vi "Process Mouse Move.vi"(0 "FSM.Graph in":T1, 5 "Display State In":T2, 7 "Coords":T3) -> (4 "FSM.Graph out":T1, 6 "Display State Out":T2, 10 "Refresh":bool)   [LabVIEW 2020, in "FSM Editor.xctl"]
uses:
  FSM Editor.xctl
  Classes/FSM.Graph/FSM.Graph.lvclass
  Classes/FSM.Port/FSM.Port.lvclass
  Drag Mode.ctl
  D:/Development/epl-vi-lib/Koop/KObject Class/KObject.lvclass
  D:/Development/epl-tosca/LV Source/FSM Graph VIs/LV Source/Classes/FSM.Graph/FSM.Graph.lvclass
  <vilib>/Utility/miscctls.llb/LVPoint32TypeDef.ctl
  State.vi
  Data.vi
  Events.ctl
  NodeAdded.ctl
  NodeSelected.ctl
  EdgeEventData.ctl
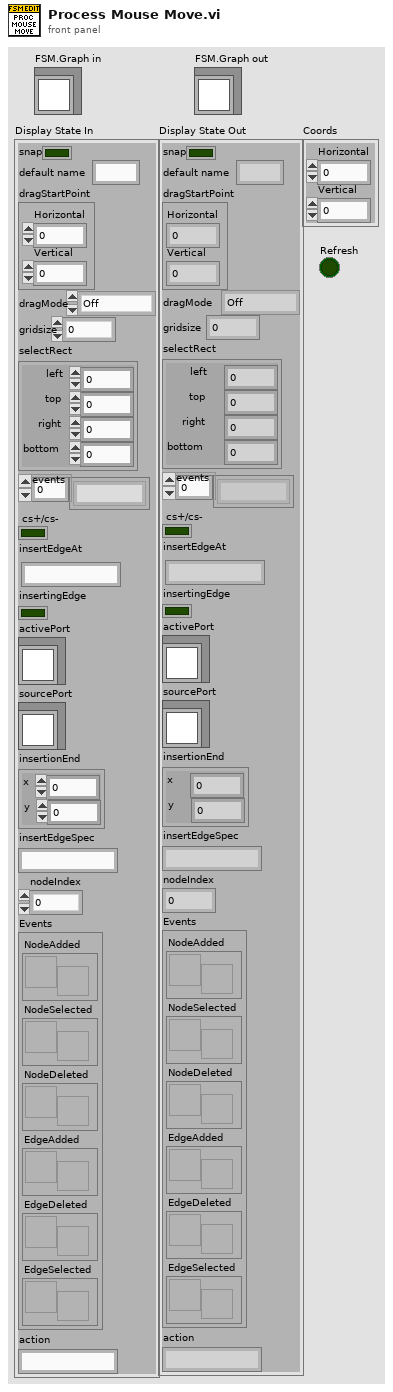
[diagram p1: front panel]
types:
  T1 = typedef "FSM Editor.xctl/Data.vi" = refnum<class "FSM.Graph.lvclass">
  T2 = typedef "FSM Editor.xctl/State.vi" = cluster{"snap":bool, "default name":string, "dragStartPoint":T3, "dragMode":T4, "gridsize":dbl, "selectRect":cluster{"left":i16, "top":i16, "right":i16, "bottom":i16}, "events":string[], "cs+/cs-":bool, "insertEdgeAt":string, "insertingEdge":bool, "activePort":refnum<class "FSM.Port.lvclass">, "sourcePort":refnum<class "FSM.Port.lvclass">, "insertionEnd":cluster{"x":i16, "y":i16}, "insertEdgeSpec":string, "nodeIndex":i32, "Events":T5, "action":string}
  T3 = typedef "LVPoint32TypeDef.ctl" = cluster{"Horizontal":i32, "Vertical":i32}
  T4 = typedef "Drag Mode.ctl" = enum16{"Off", "NodePending", "Nodes", "Pan", "Select", "EdgeInsertion", "EdgePoint", "EdgeLabel"}
  T5 = typedef "FSM Editor.xctl/Events.ctl" = cluster{"NodeAdded":refnum<user-event>, "NodeSelected":refnum<user-event>, "NodeDeleted":refnum<user-event>, "EdgeAdded":refnum<user-event>, "EdgeDeleted":refnum<user-event>, "EdgeSelected":refnum<user-event>}
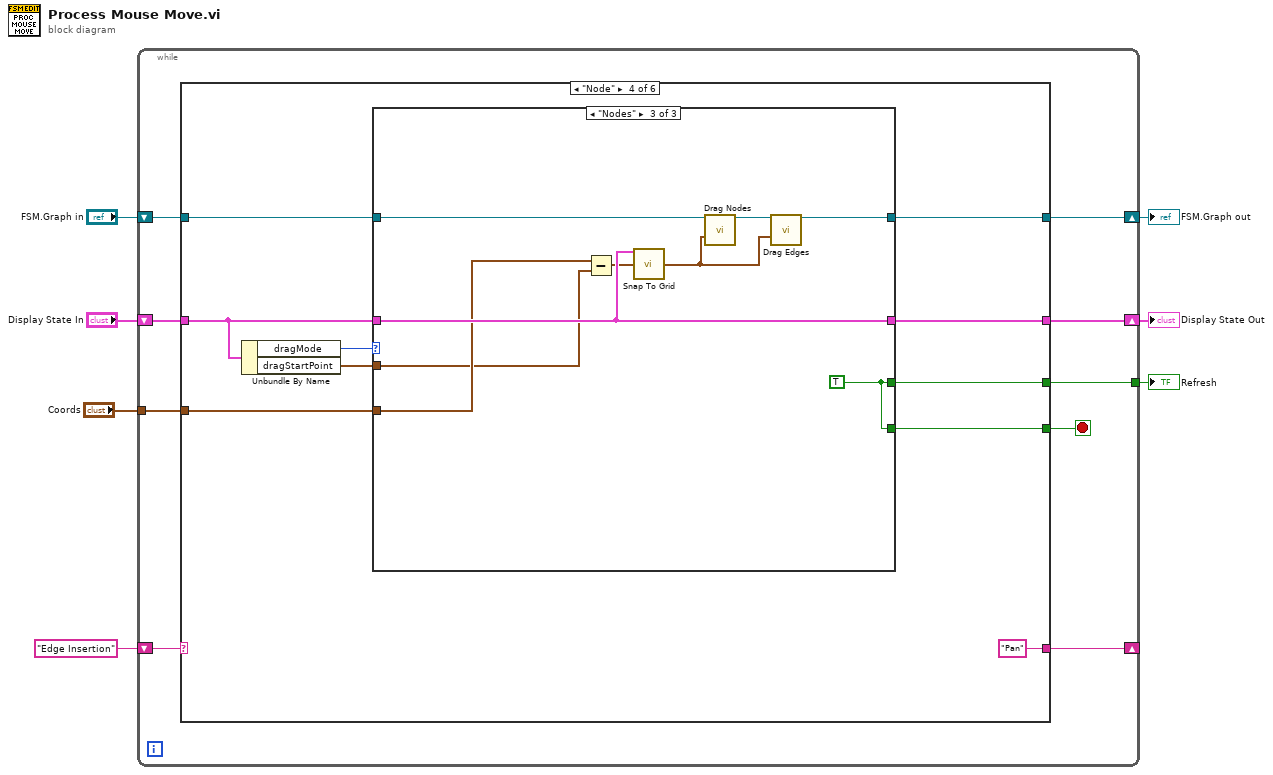
[diagram p0: block diagram]
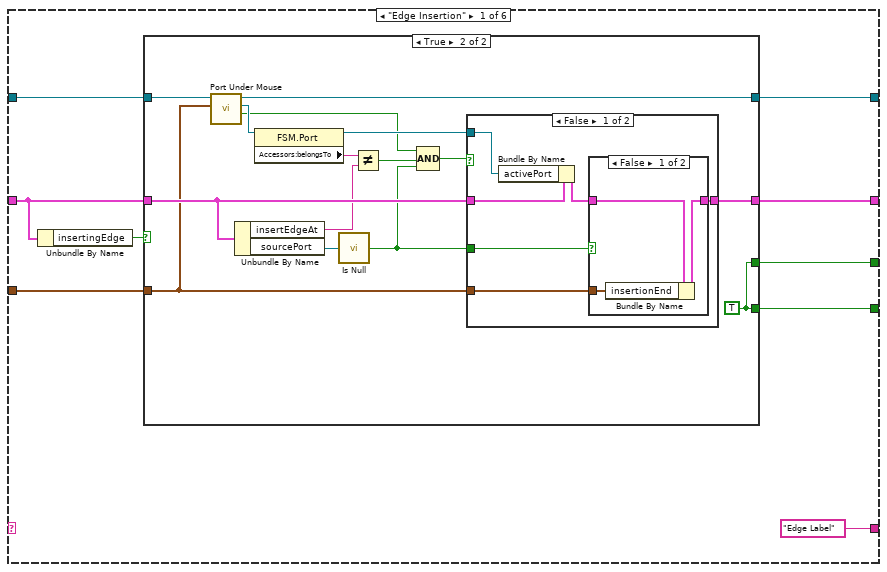
[diagram p2: hidden frame]
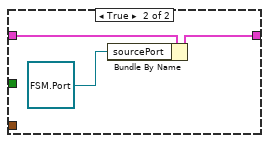
[diagram p5: hidden frame]
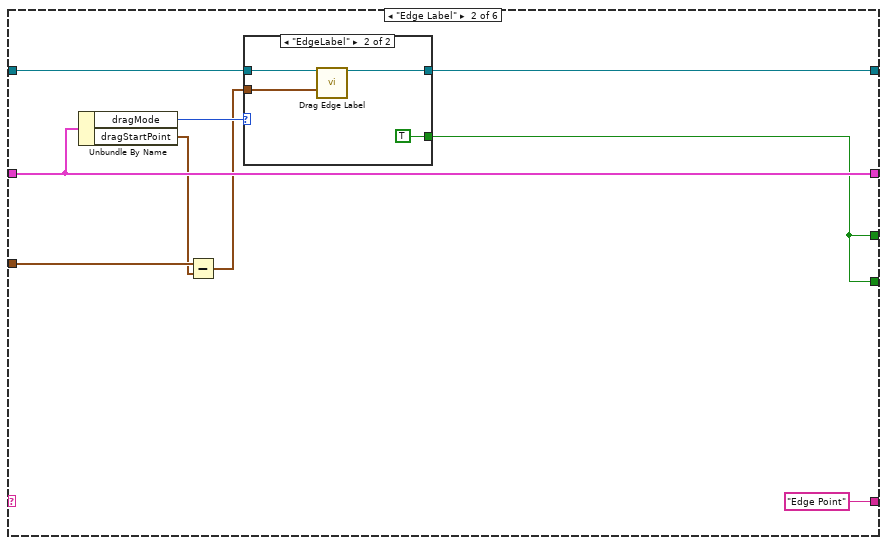
[diagram p6: hidden frame]
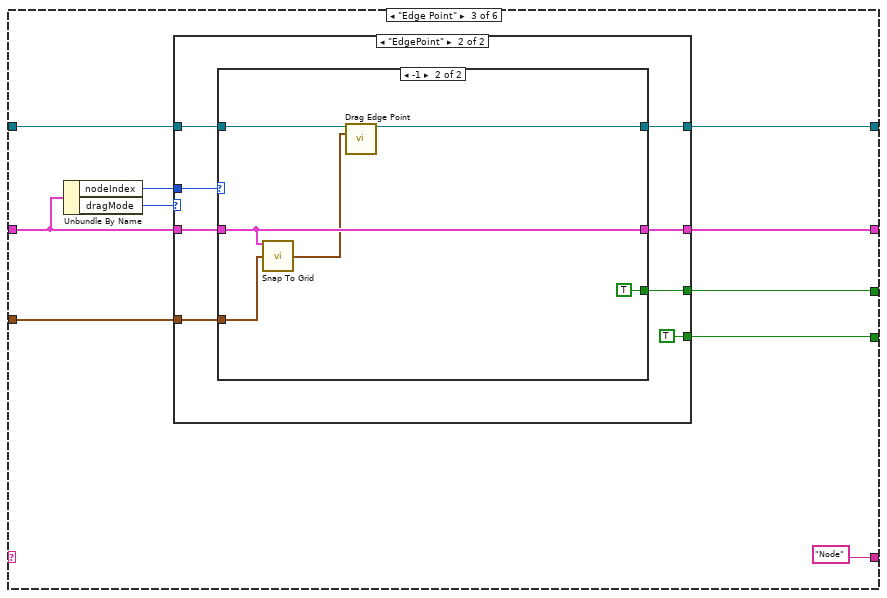
[diagram p8: hidden frame]
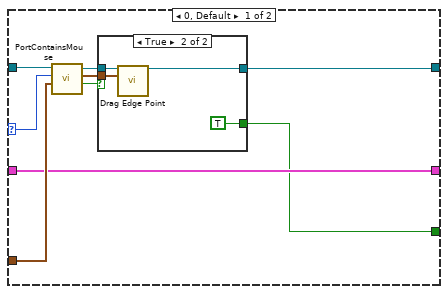
[diagram p10: hidden frame]
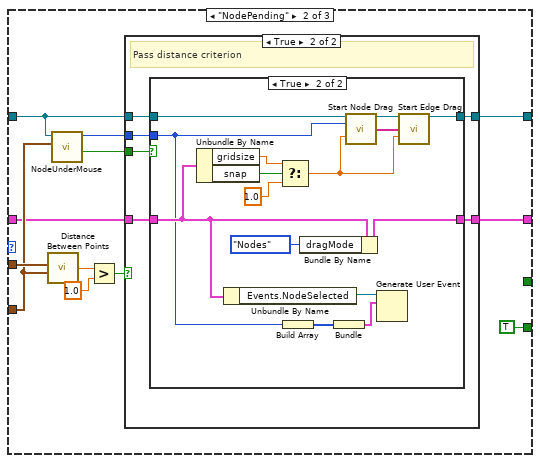
[diagram p13: hidden frame]
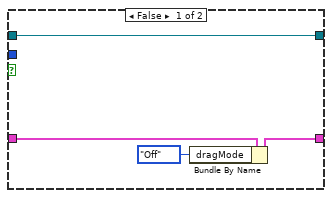
[diagram p15: hidden frame]
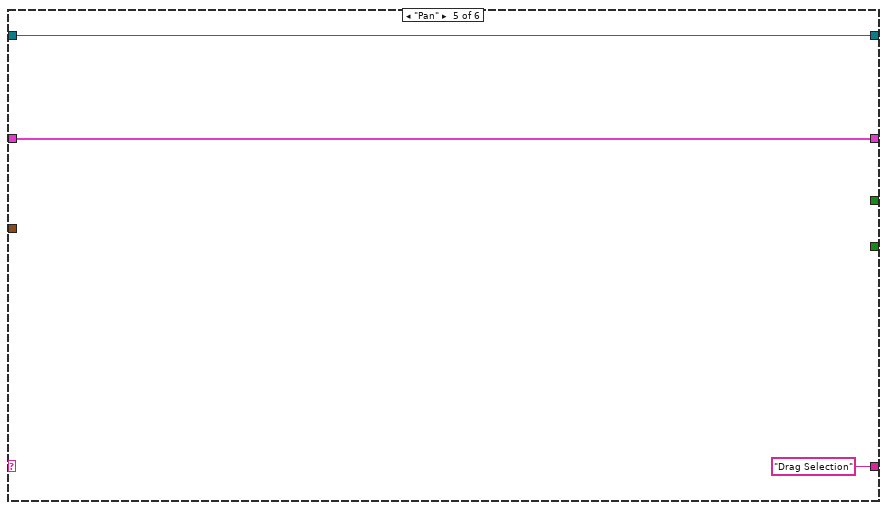
[diagram p16: hidden frame]
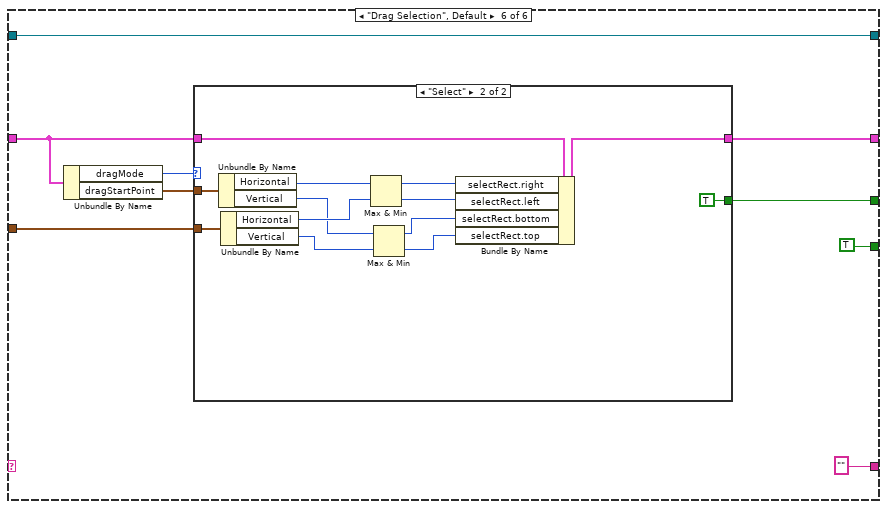
[diagram p17: hidden frame]
diagram:
  n1 = while {
    shift-right: [w14] -> w6
    shift-left: "FSM.Graph in" -> [w13]
    shift-right: [w15] -> _
    shift-left: "Edge Insertion" -> [w16]
    tunnel: "Coords" -> [w11]
    shift-right: [w10] -> w2
    shift-left: "Display State In" -> [w12]
    tunnel: [w8] -> w1
    stop <- w9 stop-if-true
    n2 = case shown="\"Node\"" w16 {
      tunnel: ["Edge Label" "Edge Point" "Node" "Pan" "Drag Selection" ""] -> w15
      tunnel: [w20 w60 w76 w116 w171 w180] -> w14
      tunnel: w13 -> [w24 w61 w77 w117 w171 w180]
      tunnel: w12 -> [w21 w63 w74 w114 w170 w178]
      tunnel: w11 -> [w23 w58 w72 w113 _ w174]
      tunnel: [w19 w63 w75 w115 w170 w176] -> w10
      tunnel: [w18 w59 w70 w110 _ TRUE] -> w9
      tunnel: [w17 w59 w71 w111 _ w173] -> w8
      frame "Edge Insertion" {
        n3 = Unbundle By Name(w21) -> ("insertingEdge"=w22:bool)
        n4 = case shown="True" w22 {
          tunnel: w24 -> [w27 w42]
          tunnel: w23 -> [_ w28]
          tunnel: w21 -> [w26 w39]
          tunnel: [w27 w40] -> w20
          tunnel: [w26 w37] -> w19
          tunnel: [_ w36] -> w18
          tunnel: [_ w36] -> w17
          frame False {
          }
          frame True {
            w36 = TRUE
            n5 = call "Port Under Mouse.vi"("point"=w28, "FSM in"=w42) -> ("found?"=w32:bool, "Port"=w41:refnum<class "FSM.Port.lvclass">, "FSM out"=w40:T1)  [unwired: 6 in, 1 out]
            n6 = Unbundle By Name(w39) -> ("insertEdgeAt"=w34:string, "sourcePort"=w30:refnum<class "FSM.Port.lvclass">)
            n7 = property class="FSM.Port"(reference=w41) -> (reference out=w38:refnum<class "FSM.Port.lvclass">, "Accessors:belongsTo"=w35:string)  [unwired: 1 in, 1 out]
            n8 = call "Is Null.vi"("Port"=w30) -> ("null"=w29:bool)
            n9 = Not Equal?(x=w35, y=w34) -> (x != y?=w33:bool)
            n10 = Compound Arithmetic op=AND(w32, w33, w29) -> (w31:bool)
            n11 = case shown="False" w31 {
              tunnel: w39 -> [w48 w55]
              tunnel: w38 -> [w47 _]
              tunnel: [w44 w54] -> w37
              tunnel: w29 -> [w46 _]
              tunnel: w28 -> [w43 _]
              frame False {
                n12 = Bundle By Name(cluster=w48, "activePort"=w47) -> (w45:T2)
                n13 = case shown="False" w46 {
                  tunnel: w45 -> [w51 w52]
                  tunnel: [w50 w52] -> w44
                  tunnel: w43 -> [w49 _]
                  frame False {
                    n14 = Bundle By Name(cluster=w51, "insertionEnd"=w49) -> (w50:T2)
                  }
                  frame True {
                  }
                }
              }
              frame True {
                n15 = Bundle By Name(cluster=w55, "sourcePort"=refnum<class "FSM.Port.lvclass"> refnum) -> (w54:T2)
              }
            }
          }
        }
      }
      frame "Edge Label" {
        n16 = Unbundle By Name(w63) -> ("dragMode"=w62:T4, "dragStartPoint"=w57:T3)
        n17 = Subtract(x=w58, y=w57) -> (x-y=w56:T3)
        n18 = case shown="\"EdgeLabel\"" w62 {
          tunnel: w61 -> [w65 w68]
          tunnel: [w65 w67] -> w60
          tunnel: [_ TRUE] -> w59
          tunnel: w56 -> [_ w66]
          frame "Off", Default {
          }
          frame "EdgeLabel" {
            n19 = call "Drag Edge Label.vi"("FSM.Graph In"=w68, "delta"=w66) -> ("FSM.Graph Out"=w67:T1)  [unwired: 13 in]
          }
        }
      }
      frame "Edge Point" {
        n20 = Unbundle By Name(w74) -> ("nodeIndex"=w73:i32, "dragMode"=w78:T4)
        n21 = case shown="\"EdgePoint\"" w78 {
          tunnel: w77 -> [w81 w88]
          tunnel: [w81 w87] -> w76
          tunnel: [w80 w85] -> w75
          tunnel: w74 -> [w80 w86]
          tunnel: w73 -> [_ w89]
          tunnel: w72 -> [_ w84]
          tunnel: [_ w83] -> w71
          tunnel: [_ TRUE] -> w70
          frame "Off", Default {
          }
          frame "EdgePoint" {
            n22 = case shown="-1" w89 {
              selector: w89 -> [w97 _]
              tunnel: w88 -> [w98 w109]
              tunnel: [w94 w108] -> w87
              tunnel: w86 -> [w93 w106]
              tunnel: [w93 w106] -> w85
              tunnel: w84 -> [w96 w105]
              tunnel: [w90 TRUE] -> w83
              frame 0, Default {
                n23 = call "PortContainsMouse.vi"("Coords"=w96, "nodeIndex"=w97, "FSM in"=w98) -> ("contains mouse"=w91:bool, "Location"=w92:cluster{"x":i16, "y":i16}, "FSM thru"=w95:T1)  [unwired: 5 in, 1 out]
                n24 = case shown="True" w91 {
                  tunnel: w95 -> [w99 w103]
                  tunnel: [w99 w102] -> w94
                  tunnel: w92 -> [_ w101]
                  tunnel: [_ TRUE] -> w90
                  frame False {
                  }
                  frame True {
                    n25 = call "Drag Edge Point.vi"("FSM.Graph In"=w103, "Location"=w101) -> ("FSM.Graph Out"=w102:T1)  [unwired: 13 in]
                  }
                }
              }
              frame -1 {
                n26 = call "Snap To Grid.vi"("Display State In"=w106, "Point In"=w105) -> ("Point Out"=w104:cluster{"Horizontal":dbl, "Vertical":dbl})  [unwired: 13 in]
                n27 = call "Drag Edge Point.vi"("FSM.Graph In"=w109, "Location"=w104) -> ("FSM.Graph Out"=w108:T1)  [unwired: 13 in]
              }
            }
          }
        }
      }
      frame "Node" {
        n28 = Unbundle By Name(w114) -> ("dragMode"=w118:T4, "dragStartPoint"=w112:T3)
        n29 = case shown="\"Nodes\"" w118 {
          tunnel: w117 -> [w121 w127 w166]
          tunnel: [w121 w124 w163] -> w116
          tunnel: [w120 w125 w169] -> w115
          tunnel: w114 -> [w120 w126 w169]
          tunnel: w113 -> [_ w132 w168]
          tunnel: w112 -> [_ w133 w167]
          tunnel: [_ _ w165] -> w111
          tunnel: [_ TRUE w165] -> w110
          frame "Off", Default {
          }
          frame "NodePending" {
            n30 = call "Distance Between Points.vi"("B"=w132, "A"=w133) -> ("distance"=w130:dbl)  [unwired: 4 in]
            n31 = call "NodeUnderMouse.vi"("Coords"=w132, "FSM in"=w127) -> ("contains mouse"=w131:bool, "Node Index"=w123:i32)  [unwired: 6 in, 2 out]
            n32 = Greater?(x=w130, y=1.0) -> (0:w128:bool)
            n33 = case shown="True" w128 {
              tunnel: w131 -> [_ w141]
              tunnel: w127 -> [w135 w140]
              tunnel: w126 -> [w134 w139]
              tunnel: [w134 w138] -> w125
              tunnel: [w135 w137] -> w124
              tunnel: w123 -> [_ w136]
              frame False {
              }
              frame True {
                # "Pass distance criterion"
                n34 = case shown="True" w141 {
                  tunnel: w140 -> [w143 w159]
                  tunnel: w139 -> [w145 w150]
                  tunnel: [w144 w160] -> w138
                  tunnel: [w143 w153] -> w137
                  tunnel: w136 -> [_ w148]
                  frame False {
                    n35 = Bundle By Name(cluster=w145, "dragMode"=Drag_Mode."Off") -> (w144:T2)
                  }
                  frame True {
                    n36 = Unbundle By Name(w150) -> ("gridsize"=w157:dbl, "snap"=w158:bool)
                    n37 = Unbundle By Name(w150) -> ("Events.NodeSelected"=w149:refnum<user-event>)
                    n38 = Select(t=w157, s=w158, f=1.0) -> (s? t:f=w152:dbl)
                    n39 = Build Array(w148) -> (w147:i32[])
                    n40 = Bundle By Name(cluster=w150, "dragMode"=Drag_Mode."Nodes") -> (w160:T2)
                    n41 = Bundle(w147) -> (w146:cluster{i32[]})  [unwired: 1 in]
                    n42 = call "Start Node Drag.vi"("FSM in"=w159, "Node index"=w148, "Grid size"=w152) -> ("FSM out"=w155:T1, "dragged nodes"=w154:string[])  [unwired: 10 in, 1 out]
                    n43 = Generate User Event(user event=w149, event data cluster=w146) -> ()  [unwired: 2 in, 2 out]
                    n44 = call "Start Edge Drag.vi"("FSM in"=w155, "Dragged nodes"=w154, "Grid size"=w152) -> ("FSM out"=w153:T1)  [unwired: 11 in, 1 out]
                  }
                }
              }
            }
          }
          frame "Nodes" {
            w165 = TRUE
            n45 = Subtract(x=w168, y=w167) -> (x-y=w162:T3)
            n46 = call "Snap To Grid.vi"("Display State In"=w169, "Point In"=w162) -> ("Point Out"=w161:cluster{"Horizontal":dbl, "Vertical":dbl})  [unwired: 13 in]
            n47 = call "Drag Nodes.vi"("FSM in"=w166, "delta"=w161) -> ("FSM out"=w164:T1)  [unwired: 11 in, 2 out]
            n48 = call "Drag Edges.vi"("FSM in"=w164, "delta"=w161) -> ("FSM out"=w163:T1)  [unwired: 12 in, 1 out]
          }
        }
      }
      frame "Pan" {
      }
      frame "Drag Selection", Default {
        n49 = Unbundle By Name(w178) -> ("dragMode"=w177:T4, "dragStartPoint"=w175:T3)
        n50 = case shown="\"Select\"" w177 {
          tunnel: w178 -> [w182 w195]
          tunnel: [w182 w188] -> w176
          tunnel: w175 -> [_ w194]
          tunnel: w174 -> [_ w192]
          tunnel: [_ TRUE] -> w173
          frame "Off", Default {
          }
          frame "Select" {
            n51 = Unbundle By Name(w194) -> ("Horizontal"=w193:i32, "Vertical"=w189:i32)
            n52 = Unbundle By Name(w192) -> ("Horizontal"=w191:i32, "Vertical"=w190:i32)
            n53 = Max & Min(x=w193, y=w191) -> (max(x,y)=w187:i32, min(x,y)=w186:i32)
            n54 = Max & Min(x=w189, y=w190) -> (max(x,y)=w185:i32, min(x,y)=w184:i32)
            n55 = Bundle By Name(cluster=w195, "selectRect.right"=w187, "selectRect.left"=w186, "selectRect.bottom"=w185, "selectRect.top"=w184) -> (w188:T2)
          }
        }
      }
    }
  }
  "Display State Out" <- w2
  "FSM.Graph out" <- w6
  "Refresh" <- w1
